vi "Set Density.vi"(7 "Density Value":i32, 8 "error in (no error)":errorcluster, 11 "Comport":refnum<visa-resource-name>) -> (0 "error out":errorcluster, 2 "Set Success":bool, 3 "Comport 2":refnum<visa-resource-name>)   [LabVIEW 2018]
panel:
  out "output array":i16[](array[numeric])
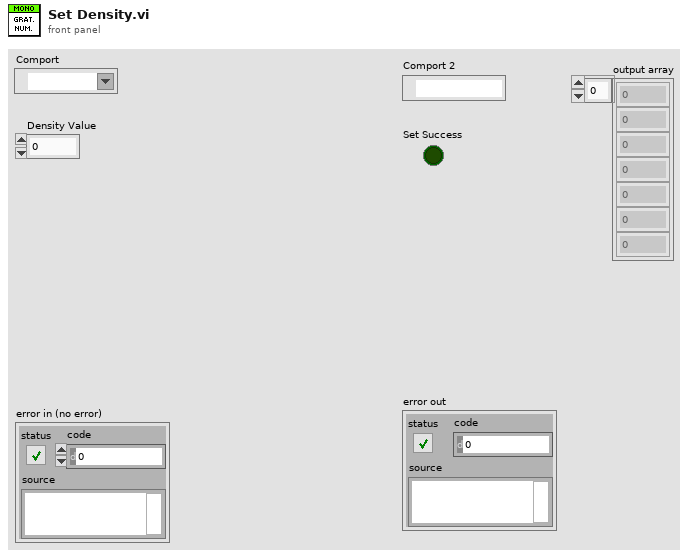
[diagram p1: front panel]
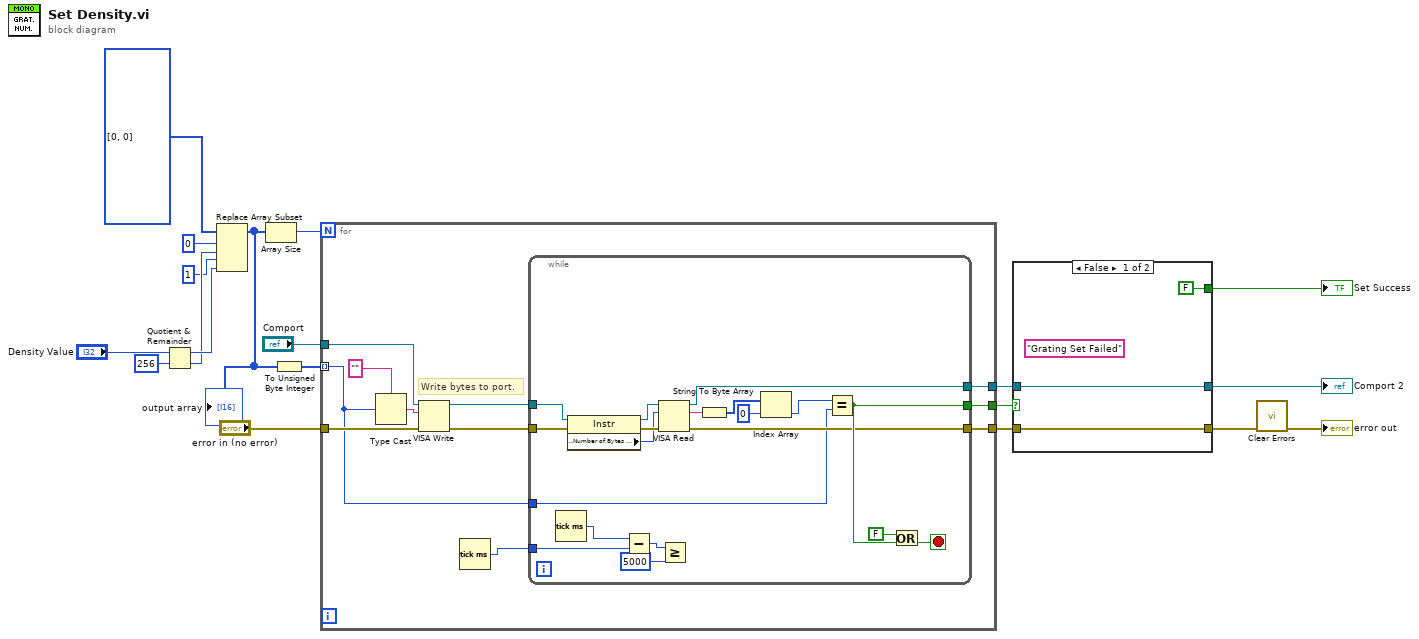
[diagram p0: block diagram]
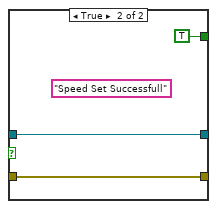
[diagram p2: hidden frame]
diagram:
  n1 = Quotient & Remainder(x="Density Value", y=u32 256) -> (x-y*floor(x/y)=w15:u32, floor(x/y)=w14:u32)
  n2 = Replace Array Subset(array=i16[] [0, 0], new element #1=w14, index #1=0 ("index"), new element #2=w15, index #2=1 ("index")) -> (w12:i16[])
  "output array" <- w12
  n3 = Array Size(array=w12) -> (size(s)=w6:i32)
  n4 = To Unsigned Byte Integer(number=w12) -> (unsigned 8bit integer=w2:u8[])
  n5 = for {
    N: w6 -> [_]
    tunnel: w2 -> [w21] mode=indexing
    tunnel: [w26] -> w7
    tunnel: [w25] -> w5
    tunnel: [w24] -> w4
    tunnel: "Comport" -> [w23]
    tunnel: "error in (no error)" -> [w22]
    # "Write bytes to port."
    n6 = Type Cast(type="", x=w21) -> (*(type *) &x=w29:string)
    n7 = VISA Write(VISA resource name=w23, write buffer=w29, error in (no error)=w22) -> (VISA resource name out=w28:refnum<visa-resource-name>, error out=w27:errorcluster)  [unwired: 1 out]
    n8 = Tick Count (ms)() -> (millisecond timer value=w20:u32)
    n9 = while {
      tunnel: w28 -> [w42]
      tunnel: w27 -> [w41]
      tunnel: [w45] -> w26
      tunnel: [w44] -> w25
      tunnel: [w43] -> w24
      tunnel: w21 -> [w37]
      tunnel: w20 -> [w35]
      stop <- w32 stop-if-true
      n10 = Tick Count (ms)() -> (millisecond timer value=w36:u32)
      n11 = property class="Instr"(reference=w42, error in=w41) -> (reference out=w40:refnum<visa-resource-name>, error out=w39:errorcluster, "Serial Settings:Number of Bytes at Serial Port"=w38:u32)
      n12 = Subtract(x=w36, y=w35) -> (x-y=w34:u32)
      n13 = VISA Read(VISA resource name=w40, byte count=w38, error in (no error)=w39) -> (VISA resource name out=w44:refnum<visa-resource-name>, read buffer=w49:string, error out=w43:errorcluster)  [unwired: 1 out]
      n14 = Greater Or Equal?(x=w34, y=u32 5000) -> ()  [unwired: 1 out]
      n15 = String To Byte Array(string=w49) -> (unsigned byte array=w48:u8[])
      n16 = Index Array(array=w48, index=0) -> (element=w46:u8)
      n17 = Equal?(x=w46, y=w37) -> (x = y?=w45:bool)
      n18 = Or(x=FALSE, y=w45) -> (x .or. y?=w32:bool)
    }
  }
  n19 = case shown="False" w7 {
    tunnel: [FALSE TRUE] -> w8
    tunnel: w5 -> [w51 w54]
    tunnel: w4 -> [w50 w53]
    tunnel: [w51 w54] -> w18
    tunnel: [w50 w53] -> w17
    frame False {
      (unwired) "Grating Set Failed" ("message")
    }
    frame True {
      (unwired) "Speed Set Successfull" ("message")
    }
  }
  "Comport 2" <- w18
  "Set Success" <- w8
  n20 = call <vilib>:"Clear Errors.vi"("error in (no error)"=w17) -> ("error out"=→"error out":errorcluster)  [unwired: 5 in, 1 out]
